vi "Ring-to-enum.vi"(11 "Set_Channel_Relay":T3 {"Relay_CH_Array"."OUTPUT_Relay_Channels" items=["CONN_SUPPLY_%d_FCT", "HB_CONN_%d_FCT", "L_IND_CONN_%d_FCT", "R_IND_CONN_%d_FCT", "SW1_%d_FCT", "SW2_%d_FCT", "CAN_H_%d_FCT", "CAN_L_%d_FCT", "CYLINDER_ON/OFF_%d_FCT", "SPARE_1_%d_FCT", "SPARE_2_%d_FCT", "Tower Red", "Tower Amber", "Tower Green", "Tower Buzzer", "SLIMRELAY_DUT_%d_FCT", "GND_DMM_%d_EOL", "CAN_H_RES_%d_EOL", "CAN_L_RES_%d_EOL", "L_IND_RES_%d_EOL", "R_IND_RES_%d_EOL", "HB_CONN_DMM_%d_EOL", "14V_RES_%d_EOL", "CAN_L_(DMM-)_%d_EOL", "CAN_H_%d_EOL", "CAN_L_%d_EOL", "14V_%d_EOL", "GND_%d_EOL", "HB_CONN_%d_EOL", "L_IND_%d_EOL", "R_IND_%d_EOL", "CYLINDER_DUT_%d_EOL", "CYL_PB_1_%d_EOL", "CYL_PB_2_%d_EOL", "DUT_PASS_%d_EOL", "DUT_FAIL_%d_EOL", "SPARE1_%d_EOL", "Tower Red_EOL", "Tower Amber_EOL", "Tower Green_EOL", "Tower Buzzer_EOL"]}) -> (3 "output cluster":T1)   [LabVIEW 2024, in "Test_2.lvlib"]
uses:
  Settings/support/Relay_Channel_Array.ctl
  Settings/support/Common_plc_DOs.ctl
  Relay_Module/support/Relay_Channel_Write.ctl
  Relay_Module/support/Relay_Enum_OUT.ctl
  Test_2.lvlib
  Relay_Module/Relay_Module.lvlib
  Settings/Setting_Screen.lvlib
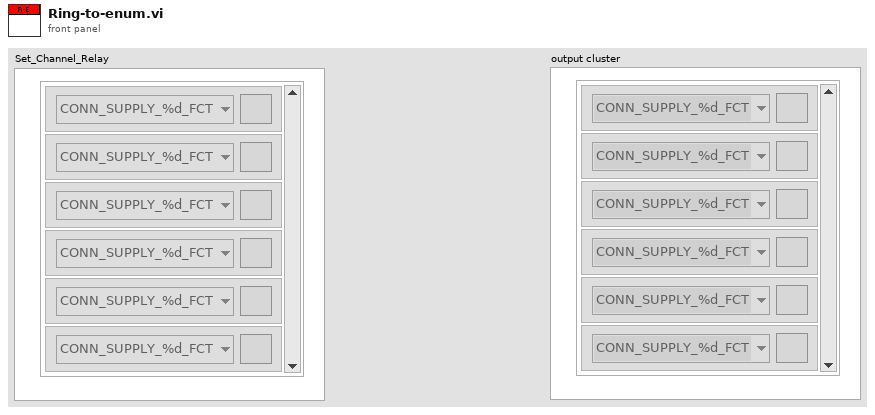
[diagram p1: front panel]
types:
  T1 = typedef "Relay_Module.lvlib/Relay_Channel_Write.ctl" = cluster{"Relay_CH_Array":cluster{"On/Off":bool, "OUTPUT_Relay_Channels":T2}[]}
  T2 = typedef "Relay_Module.lvlib/Relay_Enum_OUT.ctl" = enum16{"CONN_SUPPLY_%d_FCT", "HB_CONN_%d_FCT", "L_IND_CONN_%d_FCT", "R_IND_CONN_%d_FCT", "SW1_%d_FCT", "SW2_%d_FCT", "CAN_H_%d_FCT", "CAN_L_%d_FCT", "CYLINDER_ON/OFF_%d_FCT", "SPARE_1_%d_FCT", "SPARE_2_%d_FCT", "Tower Red", "Tower Amber", "Tower Green", "Tower Buzzer", "SLIMRELAY_DUT_%d_FCT", "GND_DMM_%d_EOL", "CAN_H_RES_%d_EOL", "CAN_L_RES_%d_EOL", "L_IND_RES_%d_EOL", "R_IND_RES_%d_EOL", "HB_CONN_DMM_%d_EOL", "14V_RES_%d_EOL", "CAN_L_(DMM-)_%d_EOL", "CAN_H_%d_EOL", "CAN_L_%d_EOL", "14V_%d_EOL", "GND_%d_EOL", "HB_CONN_%d_EOL", "L_IND_%d_EOL", "R_IND_%d_EOL", "CYLINDER_DUT_%d_EOL", "CYL_PB_1_%d_EOL", "CYL_PB_2_%d_EOL", "DUT_PASS_%d_EOL", "DUT_FAIL_%d_EOL", "SPARE1_%d_EOL", "Tower Red_EOL", "Tower Amber_EOL", "Tower Green_EOL", "Tower Buzzer_EOL"}
  T3 = typedef "Setting_Screen.lvlib/Relay_Channel_Array.ctl" = cluster{"Relay_CH_Array":cluster{"OUTPUT_Relay_Channels":T4, "On/Off":bool}[]}
  T4 = typedef "Setting_Screen.lvlib/Common_plc_DOs.ctl" = u16
  T5 = cluster{"OUTPUT_Relay_Channels":T4, "On/Off":bool}[]
  T6 = cluster{"On/Off":bool, "OUTPUT_Relay_Channels":T2}
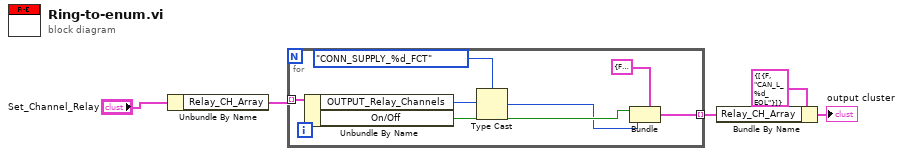
[diagram p0: block diagram]
diagram:
  n1 = Unbundle By Name("Set_Channel_Relay") -> ("Relay_CH_Array"=w4:T5)
  n2 = for {
    tunnel: w4 -> [w10] mode=indexing
    tunnel: [w6] -> w2 mode=indexing
    n3 = Unbundle By Name(w10) -> ("OUTPUT_Relay_Channels"=w12:T4, "On/Off"=w8:bool)
    n4 = Type Cast(type=Relay_Enum_OUT."CONN_SUPPLY_%d_FCT" ("OUTPUT_Relay_Channels"), x=w12) -> (*(type *) &x=w7:T2)
    n5 = Bundle(cluster=T6 {"On/Off"=FALSE, "OUTPUT_Relay_Channels"=enum."CAN_L_%d_EOL"} ("plcwrite array"), "On/Off"=w8, "OUTPUT_Relay_Channels"=w7) -> (w6:T6)
  }
  n6 = Bundle By Name(cluster=T1 {"Relay_CH_Array"=[{"On/Off"=FALSE, "OUTPUT_Relay_Channels"=enum."CAN_L_%d_EOL"}]} ("Set_Channel_Relay"), "Relay_CH_Array"=w2) -> (→"output cluster":T1)
